vi "GetChimeraResources.vi"(8 "error in (no error)":errorcluster) -> (0 "error out":errorcluster, 1 "Bitfiles":string[](array[string]), 2 "Available input channels on Automotive Camera Vision Devices":string[][](array[string]), 3 "Device Aliases":string[](array[string]))   [LabVIEW 2025, in "Automotive Vision UI.lvlib"]
doc: "Finds all available Automative Vision devices (like PXIe-1486, etc.) , filter them for those what has inputs, gathers all of the input channels, resources, types, and corresponding bitfile."
uses:
  Automotive Vision UI.lvlib
  <vilib>/nisyscfg/Filter Mode.ctl
  <vilib>/nisyscfg/nisyscfg.lvlib
  <resource>/objmgr/nicriosae.rc
  <resource>/objmgr/niflexrioatomicsae.rc
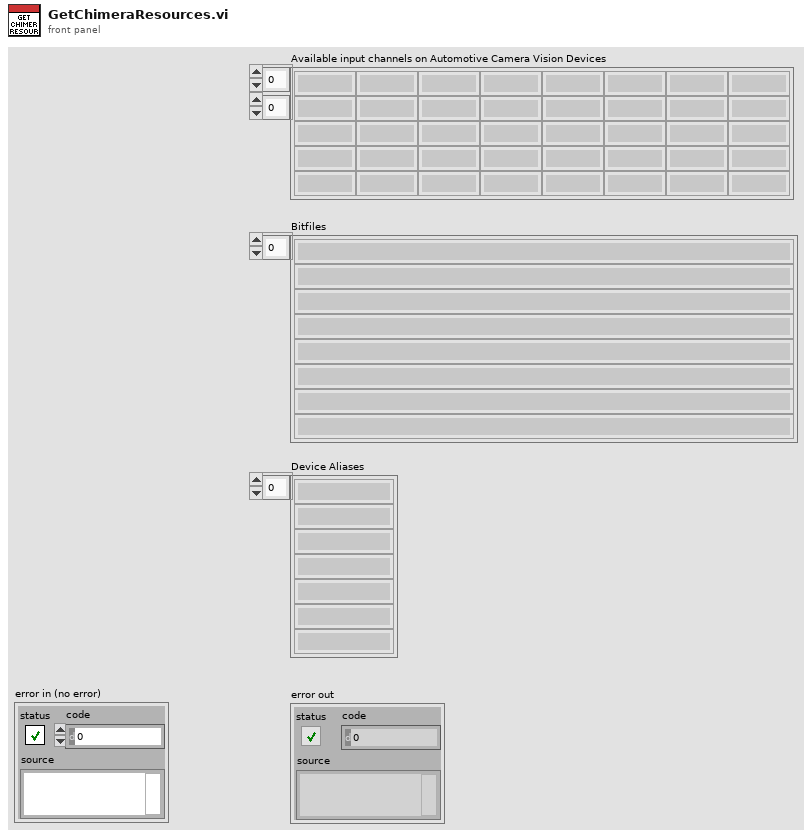
[diagram p1: front panel]
types:
  T1 = typedef "nisyscfg.lvlib/Filter Mode.ctl" = i32
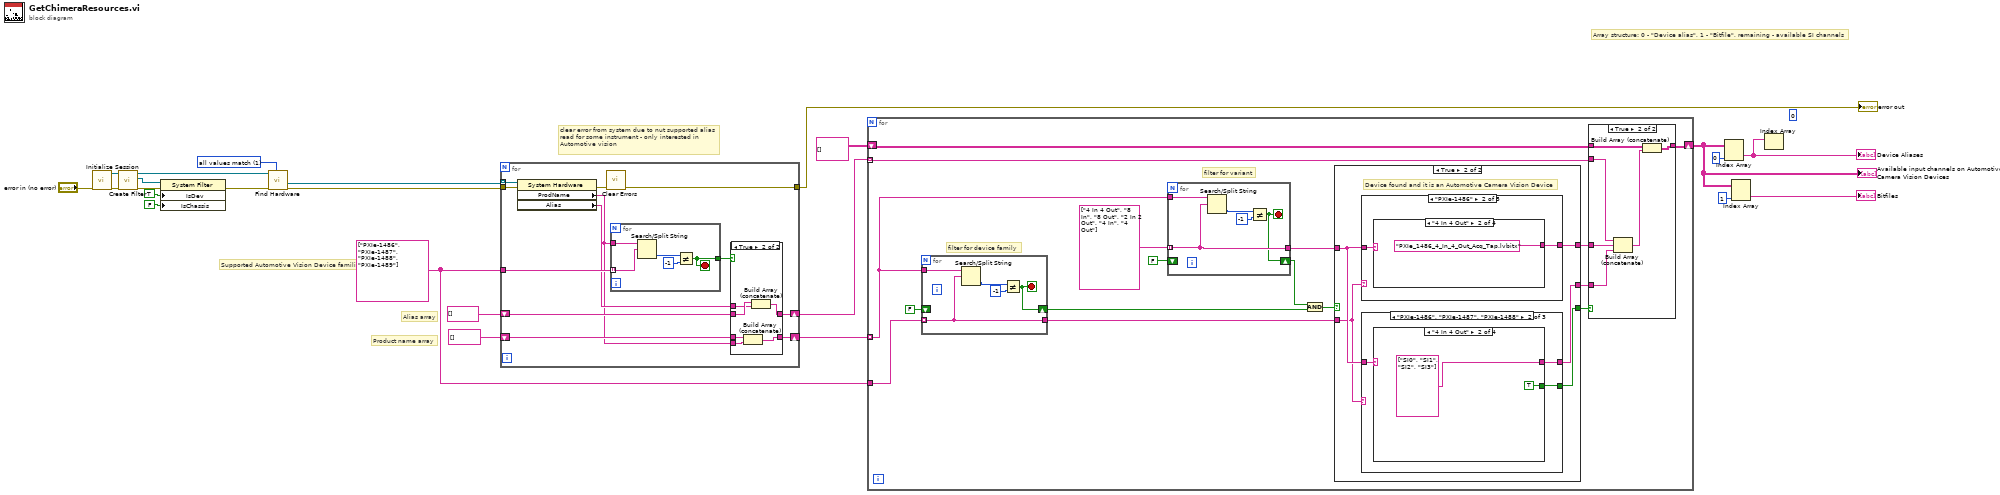
[diagram p0: block diagram]
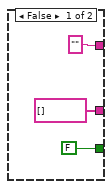
[diagram p3: hidden frame]
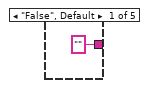
[diagram p4: hidden frame]
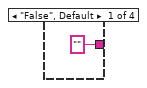
[diagram p5: hidden frame]
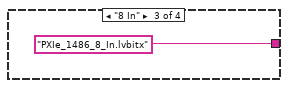
[diagram p6: hidden frame]
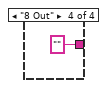
[diagram p7: hidden frame]
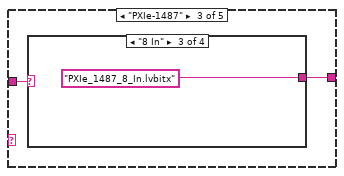
[diagram p8: hidden frame]
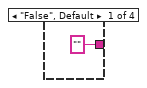
[diagram p9: hidden frame]
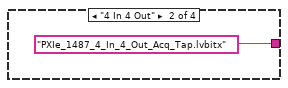
[diagram p10: hidden frame]
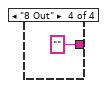
[diagram p11: hidden frame]
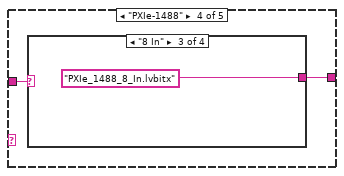
[diagram p12: hidden frame]
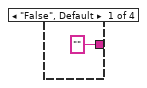
[diagram p13: hidden frame]
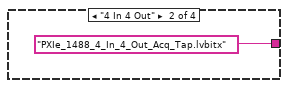
[diagram p14: hidden frame]
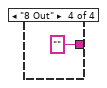
[diagram p15: hidden frame]
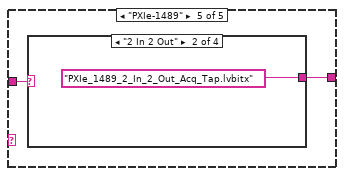
[diagram p16: hidden frame]
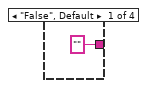
[diagram p17: hidden frame]
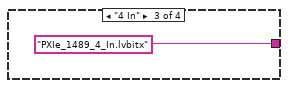
[diagram p18: hidden frame]
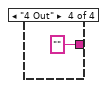
[diagram p19: hidden frame]
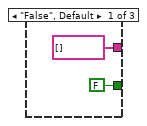
[diagram p20: hidden frame]
diagram:
  (unwired) 0
  w5 = string[] ["PXIe-1486", "PXIe-1487", "PXIe-1488", "PXIe-1489"]
  w15 = T1 1 items=["all values match"=1, "any value matches"=2, "values do not match"=3, "all properties exist"=4] ("Filter Mode (all values match)")
  # "Supported Automotive Vision Device families"
  # "clear error from system due to nut supported alias read for some instrument - only interested in Automotive vision"
  # "Array structure: 0 - \"Device alias\", 1 - \"Bitfile\", remaining - available SI channels"
  # "Product name array"
  # "Alias array"
  n1 = call <vilib>:"Initialize Session.vi"("error in (no error)"="error in (no error)") -> ("error out"=w18:errorcluster, "Session out"=w21:refnum<k21>)  [unwired: 9 in]
  n2 = call <vilib>:"Create Filter.vi"("error in (no error)"=w18, "Session in"=w21) -> ("error out"=w16:errorcluster, "Filter out"=w17:refnum<k20>, "Session out"=w22:refnum<k21>)  [unwired: 7 in]
  n3 = property on="Property Node" class="System Filter"(reference=w17, error in=w16, "IsDev"=TRUE ("Is Chassis"), "IsChassis"=FALSE ("Is Chassis")) -> (error out=w24:errorcluster)  [unwired: 1 out]
  n4 = call <vilib>:"Find Hardware.vi"("Filter Mode (all values match)"=w15, "error in (no error)"=w24, "Session in"=w22) -> ("error out"=w3:errorcluster, "Resources out"=w2:refnum<k20>[])  [unwired: 5 in, 2 out]
  n5 = for {
    tunnel: w2 -> [w35] mode=indexing
    tunnel: w5 -> [w34]
    shift-right: [w33] -> w12
    shift-left: string[] [] -> [w32]
    tunnel: w3 -> [w29]
    tunnel: [w28] -> w1
    shift-right: [w25] -> w13
    shift-left: string[] [] -> [w27]
    n6 = property on="Property Node" class="System Hardware"(reference=w35, error in=w29) -> (error out=w36:errorcluster, "ProdName"=w26:string, "Alias"=w30:string)  [unwired: 1 out]
    n7 = call <vilib>:"Clear Errors.vi"("error in (no error)"=w36) -> ("error out"=w28:errorcluster)  [unwired: 5 in, 1 out]
    n8 = for {
      tunnel: w26 -> [w49]
      tunnel: w34 -> [w48] mode=indexing
      tunnel: [w45] -> w31
      stop <- w45 stop-if-true
      n9 = Search/Split String(string=w49, search string/char (-)=w48) -> (offset of match=w47:i32)  [unwired: 1 in, 2 out]
      n10 = Not Equal?(x=w47, y=-1) -> (x != y?=w45:bool)
    }
    n11 = case shown="True" w31 {
      tunnel: [w38 w43] -> w33
      tunnel: w32 -> [w38 w44]
      tunnel: w30 -> [_ w42]
      tunnel: w27 -> [w37 w41]
      tunnel: w26 -> [_ w40]
      tunnel: [w37 w39] -> w25
      frame False {
      }
      frame True {
        n12 = Build Array (concatenate)(w41, w40) -> (w39:string[])
        n13 = Build Array (concatenate)(w44, w42) -> (w43:string[])
      }
    }
  }
  "error out" <- w1
  n14 = for {
    tunnel: w13 -> [w50] mode=indexing
    tunnel: w12 -> [w57] mode=indexing
    shift-right: [w53] -> w9
    shift-left: string[][] [] -> [w52]
    tunnel: w5 -> [w51]
    # "filter for variant"
    # "filter for device family"
    n15 = for {
      tunnel: w50 -> [w82]
      tunnel: w51 -> [w79] mode=indexing
      tunnel: [w79] -> w62
      shift-right: [w78] -> w60
      shift-left: FALSE -> [_]
      stop <- w78 stop-if-true
      n16 = Search/Split String(string=w82, search string/char (-)=w79) -> (offset of match=w80:i32)  [unwired: 1 in, 2 out]
      n17 = Not Equal?(x=w80, y=-1) -> (x != y?=w78:bool)
    }
    n18 = for {
      tunnel: w50 -> [w77]
      tunnel: string[] ["4 In 4 Out", "8 In", "8 Out", "2 In 2 Out", "4 In", "4 Out"] -> [w74] mode=indexing
      tunnel: [w74] -> w58
      shift-right: [w73] -> w61
      shift-left: FALSE -> [_]
      stop <- w73 stop-if-true
      n19 = Search/Split String(string=w77, search string/char (-)=w74) -> (offset of match=w75:i32)  [unwired: 1 in, 2 out]
      n20 = Not Equal?(x=w75, y=-1) -> (x != y?=w73:bool)
    }
    n21 = And(x=w61, y=w60) -> (x .and. y?=w59:bool)
    n22 = case shown="True" w59 {
      tunnel: w62 -> [_ w87]
      tunnel: w58 -> [_ w88]
      tunnel: [string[] [] w90] -> w56
      tunnel: [FALSE w89] -> w55
      tunnel: ["" w86] -> w54
      frame False {
      }
      frame True {
        # "Device found and it is an Automotive Camera Vision Device"
        n23 = case shown="\"PXIe-1486\", \"PXIe-1487\", \"PXIe-1488\"" w87 {
          tunnel: w88 -> [_ w120 w131]
          tunnel: [string[] [] w119 w130] -> w90
          tunnel: [FALSE w118 w129] -> w89
          frame "False", Default {
          }
          frame "PXIe-1486", "PXIe-1487", "PXIe-1488" {
            n24 = case shown="\"4 In 4 Out\"" w120 {
              tunnel: [string[] [] string[] ["SI0", "SI1", "SI2", "SI3"] string[] ["SI0", "SI1", "SI2", "SI3", "SI4", "SI5", "SI6", "SI7"] string[] []] -> w119
              tunnel: [FALSE TRUE TRUE FALSE] -> w118
              frame "False", Default {
              }
              frame "4 In 4 Out" {
              }
              frame "8 In" {
              }
              frame "8 Out" {
              }
            }
          }
          frame "PXIe-1489" {
            n25 = case shown="\"False\", Default" w131 {
              tunnel: [string[] [] string[] ["SI0", "SI1"] string[] ["SI0", "SI1", "SI2", "SI3"] string[] []] -> w130
              tunnel: [FALSE TRUE TRUE FALSE] -> w129
              frame "False", Default {
              }
              frame "2 In 2 Out" {
              }
              frame "4 In" {
              }
              frame "4 Out" {
              }
            }
          }
        }
        n26 = case shown="\"PXIe-1486\"" w87 {
          tunnel: ["" w93 w99 w105 w111] -> w86
          tunnel: w88 -> [_ w92 w98 w104 w110]
          frame "False", Default {
          }
          frame "PXIe-1486" {
            n27 = case shown="\"4 In 4 Out\"" w92 {
              tunnel: ["" "PXIe_1486_4_In_4_Out_Acq_Tap.lvbitx" "PXIe_1486_8_In.lvbitx" ""] -> w93
              frame "False", Default {
              }
              frame "4 In 4 Out" {
              }
              frame "8 In" {
              }
              frame "8 Out" {
              }
            }
          }
          frame "PXIe-1487" {
            n28 = case shown="\"8 In\"" w98 {
              tunnel: ["" "PXIe_1487_4_In_4_Out_Acq_Tap.lvbitx" "PXIe_1487_8_In.lvbitx" ""] -> w99
              frame "False", Default {
              }
              frame "4 In 4 Out" {
              }
              frame "8 In" {
              }
              frame "8 Out" {
              }
            }
          }
          frame "PXIe-1488" {
            n29 = case shown="\"8 In\"" w104 {
              tunnel: ["" "PXIe_1488_4_In_4_Out_Acq_Tap.lvbitx" "PXIe_1488_8_In.lvbitx" ""] -> w105
              frame "False", Default {
              }
              frame "4 In 4 Out" {
              }
              frame "8 In" {
              }
              frame "8 Out" {
              }
            }
          }
          frame "PXIe-1489" {
            n30 = case shown="\"2 In 2 Out\"" w110 {
              tunnel: ["" "PXIe_1489_2_In_2_Out_Acq_Tap.lvbitx" "PXIe_1489_4_In.lvbitx" ""] -> w111
              frame "False", Default {
              }
              frame "2 In 2 Out" {
              }
              frame "4 In" {
              }
              frame "4 Out" {
              }
            }
          }
        }
      }
    }
    n31 = case shown="True" w55 {
      tunnel: w57 -> [_ w72]
      tunnel: w56 -> [_ w70]
      tunnel: w54 -> [_ w71]
      tunnel: [w66 w68] -> w53
      tunnel: w52 -> [w66 w69]
      frame False {
      }
      frame True {
        n32 = Build Array (concatenate)(w72, w71, w70) -> (w67:string[])
        n33 = Build Array (concatenate)(w69, w67) -> (w68:string[][])
      }
    }
  }
  "Available input channels on Automotive Camera Vision Devices" <- w9
  n34 = Index Array(array=w9, index (col)=0 ("disabled index (col)")) -> (element=w6:string[])  [unwired: 1 in]
  "Device Aliases" <- w6
  n35 = Index Array(array=w9, index (col)=1 ("disabled index (col)")) -> (element=→"Bitfiles":string[])  [unwired: 1 in]
  n36 = Index Array(array=w6) -> ()  [unwired: 1 in, 1 out]
